vi "Connection Mode Generation Create New TP Connection.vi"(2 "Allow Any SA":bool=TRUE, 5 "Data to Send":T1 {"Identifier" format="%08x"}, 7 "Source Address":u8, 11 "error in (no error)":errorcluster) -> (4 "Connections Cluster":T2 {"Packets"."Identifier" format="%08x"}, 6 "Connection Management Packet":T1 {"Identifier" format="%08x"}, 15 "error out":errorcluster)   [LabVIEW 2013, in "J1939.lvlib"]
uses:
  J1939.lvlib
  Connection Mode Generation Connection Cluster.ctl
  API Types/CAN Outgoing Message Cluster.ctl
  Frame Conversion/Convert CAN Arb ID to J1939 ID.vi
  Common Messages/J1939 Message TP.CM RTS.vi
  Common Messages/J1939 Message TP.DT.vi
  Frame Conversion/Convert J1939 ID to CAN Arb ID.vi
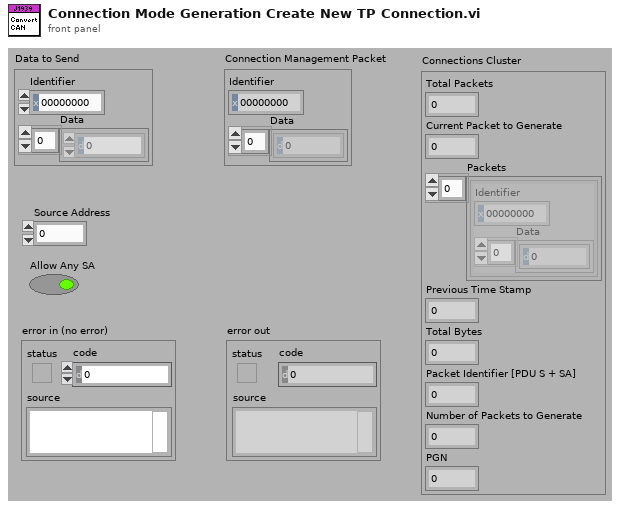
[diagram p1: front panel]
types:
  T1 = typedef "J1939.lvlib/CAN Outgoing Message Cluster.ctl" = cluster{"Identifier":u32, "Data":u8[]}
  T2 = typedef "J1939.lvlib/Connection Mode Generation Connection Cluster.ctl" = cluster{"Total Packets":u8, "Current Packet to Generate":u8, "Packets":T1[], "Previous Time Stamp":u32, "Total Bytes":u16, "Packet Identifier [PDU S + SA]":u16, "Number of Packets to Generate":u8, "PGN":u32}
  T3 = typedef "J1939.lvlib/PGN Fields Cluster.ctl" = cluster{"Reserved Bit":u8, "Data page":u8, "PDU Format":u8, "PDU Specific":u8}
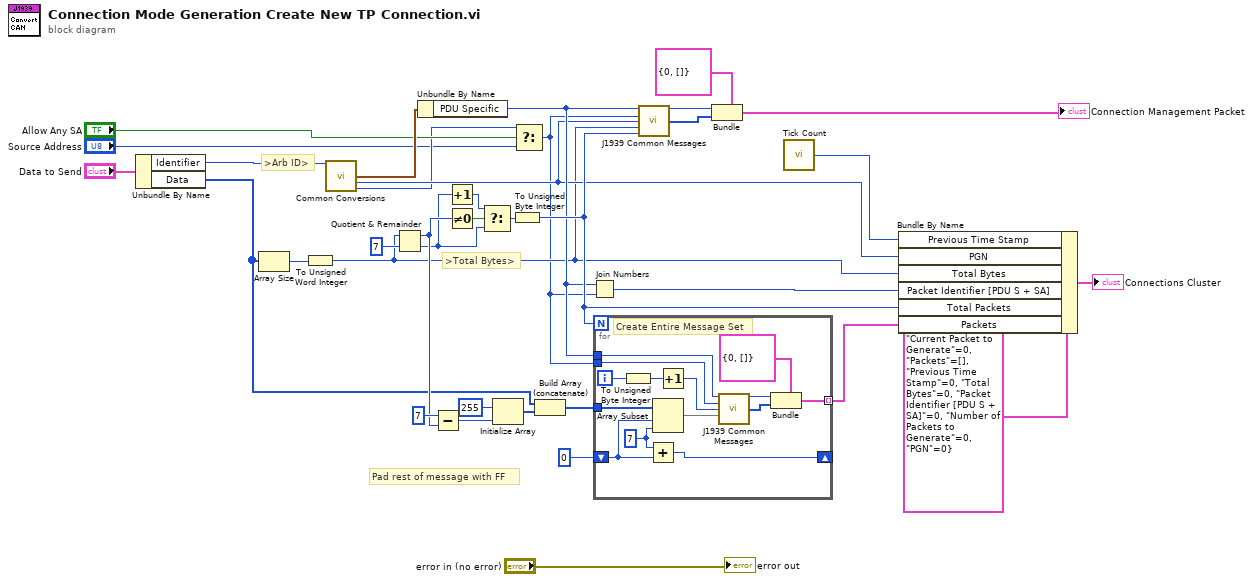
[diagram p0: block diagram]
diagram:
  # "Pad rest of message with FF"
  # ">Arb ID>"
  # ">Total Bytes>"
  n1 = Unbundle By Name("Data to Send") -> ("Identifier"=w12:u32, "Data"=w5:u8[])
  n2 = Array Size(array=w5) -> (size(s)=w17:i32)
  n3 = To Unsigned Word Integer(number=w17) -> (unsigned 16bit integer=w6:u16)
  n4 = call-poly "Common Conversions.vi"("Arb ID"=w12) -> ("PGN Fields"=w34:T3, "PGN"=w16:u32, "Source Address"=w3:u8)  [unwired: 12 out]
  n5 = Quotient & Remainder(x=w6, y=u16 7) -> (x-y*floor(x/y)=w28:u16, floor(x/y)=w24:u16)
  n6 = Unbundle By Name(w34) -> ("PDU Specific"=w18:u8)
  n7 = Subtract(x=u8 7, y=w28) -> (x-y=w30:u16)
  n8 = Increment(x=w24) -> (x+1=w23:u16)
  n9 = Not Equal To 0?(x=w28) -> (x != 0?=w22:bool)
  n10 = Select(t=w23, s=w22, f=w24) -> (s? t:f=w25:u16)
  n11 = Initialize Array(u8 255, w30) -> (w31:u8[])
  n12 = To Unsigned Byte Integer(number=w25) -> (unsigned 8bit integer=w19:u8)
  n13 = Select(t=w3, s="Allow Any SA", f="Source Address") -> (s? t:f=w1:u8)
  n14 = Build Array (concatenate)(w5, w31) -> (w32:u8[])
  n15 = Join Numbers(hi=w18, lo=w1) -> ((hi.lo)=w35:u16)
  n16 = for {
    N: w19 -> [_]
    tunnel: w32 -> [w49]
    shift-right: [w46] -> _
    shift-left: 0 ("index") -> [w47]
    tunnel: [w37] -> w11 mode=indexing
    tunnel: w1 -> [w42]
    tunnel: w18 -> [w43]
    i -> [w45]
    w48 = 7 ("length")
    # "Create Entire Message Set"
    n17 = To Unsigned Byte Integer(number=w45) -> (unsigned 8bit integer=w44:u8)
    n18 = Add(x=w48, y=w47) -> (x+y=w46:i32)
    n19 = Array Subset(array=w49, index=w47, length=w48) -> (w40:u8[])
    n20 = Increment(x=w44) -> (x+1=w41:u8)
    n21 = call-poly "J1939 Common Messages.vi"("Destination Address"=w43, "Source Address"=w42, "Sequence Number"=w41, "Data"=w40) -> ("Arb ID"=w39:u32, "Data"=w38:u8[])  [unwired: 10 out]
    n22 = Bundle(cluster=T1 {"Identifier"=0, "Data"=[]}, "Identifier"=w39, "Data"=w38) -> (w37:T1)
  }
  n23 = call-poly "J1939 Common Messages.vi"("Destination Address"=w18, "Source Address"=w1, "PGN"=w16, "Total Message Size(bytes)"=w6, "Total Number of Packets"=w19) -> ("Arb ID"=w15:u32, "Data"=w14:u8[])  [unwired: 9 out]
  n24 = Bundle(cluster=T1 {"Identifier"=0, "Data"=[]}, "Identifier"=w15, "Data"=w14) -> (→"Connection Management Packet":T1)
  n25 = call "Tick Count"() -> ("Tick Count(mSec)"=w8:u32)
  n26 = Bundle By Name(cluster=T2 {"Total Packets"=0, "Current Packet to Generate"=0, "Packets"=[], "Previous Time Stamp"=0, "Total Bytes"=0, "Packet Identifier [PDU S + SA]"=0, "Number of Packets to Generate"=0, "PGN"=0} ("Cluster"), "Previous Time Stamp"=w8, "PGN"=w16, "Total Bytes"=w6, "Packet Identifier [PDU S + SA]"=w35, "Total Packets"=w19, "Packets"=w11) -> (→"Connections Cluster":T2)
  "error out" <- "error in (no error)"
